vi "Generate Temperature Voltage Pairs.vi"(8 "error in (no error)":errorcluster, 11 "filenames":string[](array[string])) -> (0 "error out":errorcluster, 1 "V & T Pairs":i32, 2 "Average Temperatures":dbl[](array[numeric]), 3 "Average Voltages":dbl[][](array[numeric]))   [LabVIEW 2019, in "Analysis.lvlib"]
doc: "Message loop for handling messages pertaining to the analysis of data from the acquisition loop."
uses:
  Analysis.lvlib
panel:
  in  "data type":T1
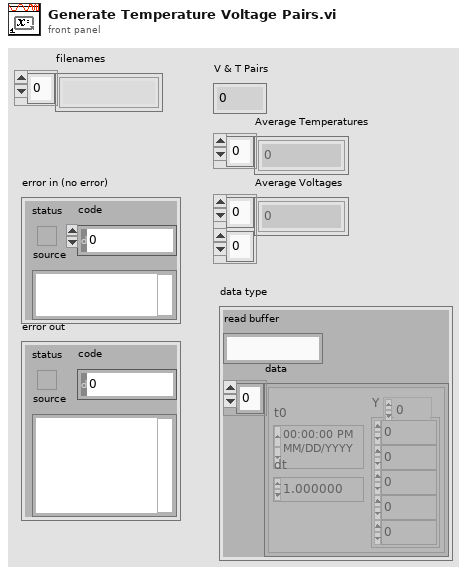
[diagram p1: front panel]
types:
  T1 = cluster{"read buffer":string, "data":waveform(dbl)[]}
  T2 = cluster{"read buffer":string, "data":waveform(dbl)[]}[]
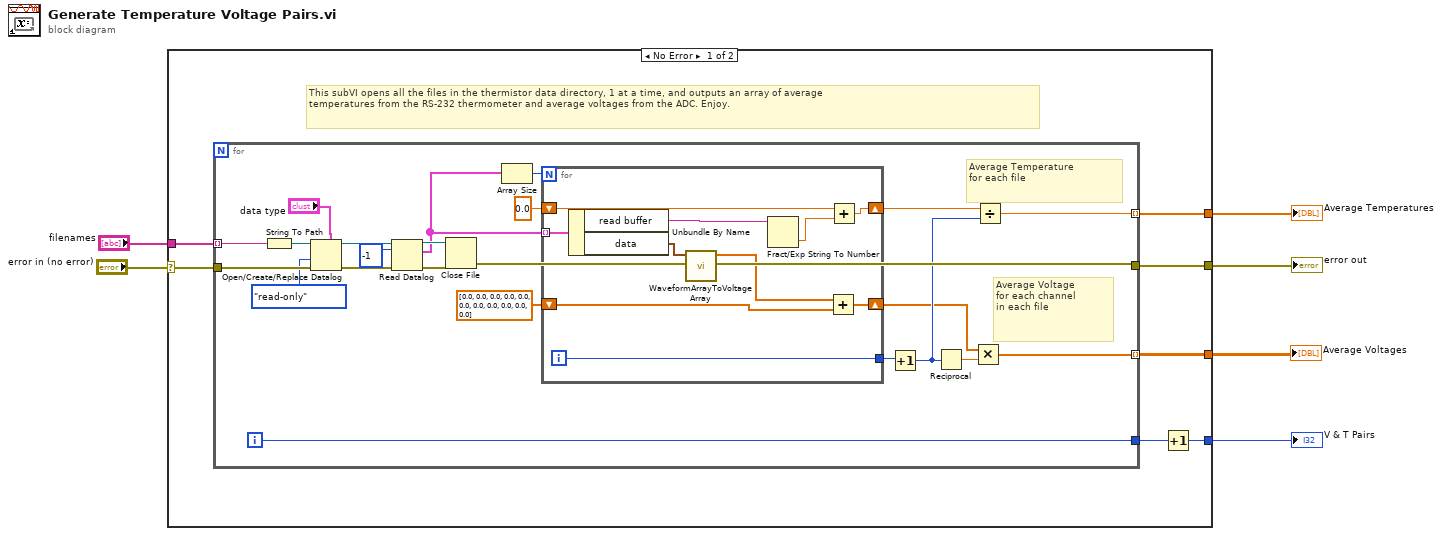
[diagram p0: block diagram]
diagram:
  n1 = case shown="No Error" "error in (no error)" {
    selector: "error in (no error)" -> [w12 w47]
    tunnel: [w7 w47] -> w6
    tunnel: "filenames" -> [w13 _]
    tunnel: [w11 _] -> w2
    tunnel: [w10 _] -> w1
    tunnel: [w9 _] -> w3
    frame No Error {
      # "This subVI opens all the files in the thermistor data directory, 1 at a time, and outputs an array of average \ntemperatures from the RS-232 thermometer and average voltages from the ADC. Enjoy."
      n2 = for {
        tunnel: w13 -> [w35] mode=indexing
        tunnel: w12 -> [w23]
        tunnel: [w30] -> w11 mode=indexing
        tunnel: [w25] -> w10 mode=indexing
        tunnel: [w29] -> w8
        tunnel: [w36] -> w7
        i -> [w29]
        # "Average Temperature\nfor each file"
        # "Average Voltage\nfor each channel\nin each file"
        n3 = String To Path(string=w35) -> (path=w24:path)
        n4 = Open/Create/Replace Datalog(5:"data type", 8:w23, 9:enum16{"read/write", "read-only", "write-only"}."read-only" ("access (0:read/write)"), 11:w24) -> (0:w20:errorcluster, 3:w16:refnum<k1>)  [unwired: 2 in, 1 out]
        n5 = Read Datalog(4:w20, 6:-1 ("count (1)"), 7:w16) -> (0:w19:errorcluster, 2:w14:T2, 3:w17:refnum<k1>)
        n6 = Close File(refnum=w17, error in=w19) -> (error out=w36:errorcluster)  [unwired: 1 out]
        n7 = Array Size(array=w14) -> (size(s)=w15:i32)
        n8 = for {
          N: w15 -> [_]
          tunnel: w14 -> [w46] mode=indexing
          shift-right: [w44] -> w31
          shift-left: 0.0 -> [w43]
          shift-right: [w40] -> w26
          shift-left: dbl[] [0.0, 0.0, 0.0, 0.0, 0.0, 0.0, 0.0, 0.0, 0.0, 0.0, 0.0] -> [w38]
          tunnel: [w37] -> w32
          i -> [w37]
          n9 = Unbundle By Name(w46) -> ("read buffer"=w45:string, "data"=w41:waveform(dbl)[])
          n10 = call "WaveformArrayToVoltageArray.vi"("Waveform Array"=w41) -> ("Average Voltage"=w39:dbl[])  [unwired: 10 in]
          n11 = Fract/Exp String To Number(string=w45) -> (number=w42:dbl)  [unwired: 3 in, 1 out]
          n12 = Add(x=w39, y=w38) -> (x+y=w40:dbl[])
          n13 = Add(x=w43, y=w42) -> (x+y=w44:dbl)
        }
        n14 = Increment(x=w32) -> (x+1=w28:i32)
        n15 = Reciprocal(x=w28) -> (1/x=w27:dbl)
        n16 = Multiply(x=w26, y=w27) -> (x*y=w25:dbl[])
        n17 = Divide(x=w31, y=w28) -> (x/y=w30:dbl)
      }
      n18 = Increment(x=w8) -> (x+1=w9:i32)
    }
    frame Error {
    }
  }
  "error out" <- w6
  "V & T Pairs" <- w3
  "Average Temperatures" <- w2
  "Average Voltages" <- w1
